vi "4461.Start.AI.vi"(6 "error in (no error)":errorcluster, 9 "Instrument.Lockin in":refnum<class "Instrument.Lockin.lvclass">) -> (0 "error out":errorcluster, 3 "Instrument.Lockin out":refnum<class "Instrument.Lockin.lvclass">)   [LabVIEW 2016, in "LockinDAQ.lvclass"]
uses:
  LockinDAQ.lvclass
  <resource>/objmgr/daqmx.rc
  <vilib>/DAQmx/read.llb/DAQmx Read (Analog 1D Wfm NChan NSamp).vi
  Instrument.Lockin/Instrument.Lockin.lvclass
  C:/Program Files (x86)/National Instruments/LabVIEW 2016/user.lib/LevyLab/Levylab Instruments/SMOs/Instrument/Instrument.lvclass
  C:/Program Files (x86)/National Instruments/LabVIEW 2016/user.lib/LevyLab/Levylab Instruments/SMOs/LevyLab/LevyLab.lvclass
  C:/Program Files (x86)/National Instruments/LabVIEW 2016/vi.lib/JKI/JKI SMO/SMO/SMO.lvclass
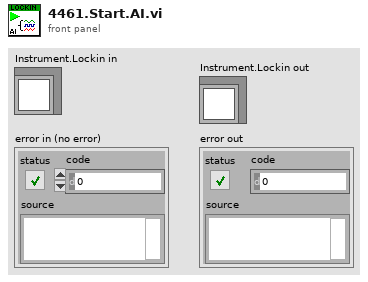
[diagram p1: front panel]
types:
  T1 = typedef "LockinDAQ.lvclass/DAQType-enum.ctl" = enum16{"None", "USB 4431", "PXI 446x"}
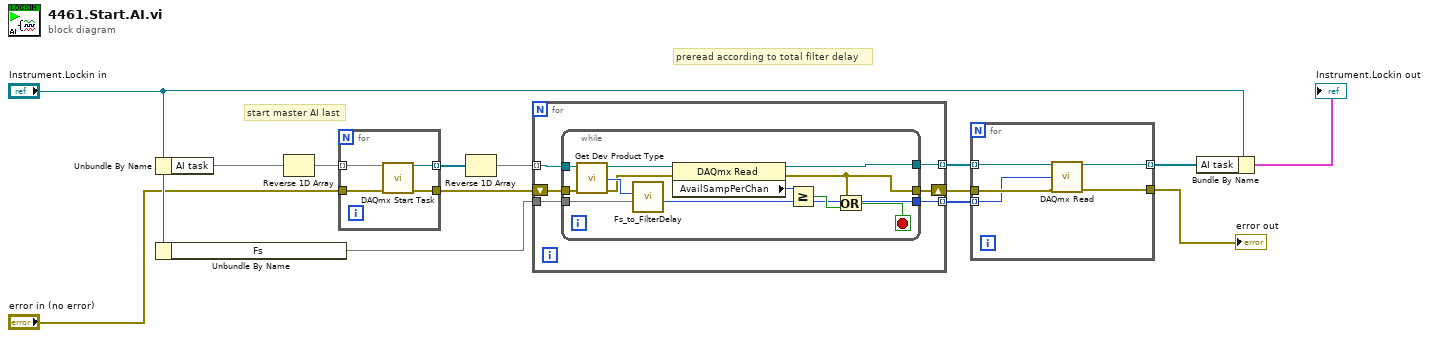
[diagram p0: block diagram]
diagram:
  # "preread according to total filter delay"
  # "start master AI last"
  n1 = Unbundle By Name("Instrument.Lockin in") -> ("AI task"=w12)
  n2 = Unbundle By Name("Instrument.Lockin in") -> ("Fs"=w8)
  n3 = Reverse 1D Array(array=w12) -> (reversed array=w11:void[])
  n4 = for {
    tunnel: w11 -> [w18] mode=indexing
    tunnel: "error in (no error)" -> [w17]
    tunnel: [w16] -> w10 mode=indexing
    tunnel: [w15] -> w9
    n5 = call <vilib>:"DAQmx Start Task.vi"("task/channels in"=w18, "error in"=w17) -> ("task out"=w16:refnum<k21>, "error out"=w15:errorcluster)  [unwired: 12 in]
  }
  n6 = Reverse 1D Array(array=w10) -> (reversed array=w1:refnum<k21>[])
  n7 = for {
    tunnel: w1 -> [w24] mode=indexing
    tunnel: w8 -> [w22]
    shift-right: [w21] -> w5
    shift-left: w9 -> [w23]
    tunnel: [w20] -> w7 mode=indexing
    tunnel: [w19] -> w6 mode=indexing
    n8 = while {
      tunnel: w24 -> [w36]
      tunnel: w23 -> [w35]
      tunnel: w22 -> [w34]
      tunnel: [w27] -> w21
      tunnel: [w26] -> w20
      tunnel: [w25] -> w19
      stop <- w29 stop-if-true
      n9 = call "Get Dev Product Type.vi"("error in (no error)"=w35, "Refnum in"=w36) -> ("error out"=w28:errorcluster, "DAQ Type"=w33:T1, "Refnum out"=w32:refnum<k21>)  [unwired: 6 in, 1 out]
      n10 = call "Fs_to_FilterDelay.vi"("Fs"=w34, "DAQ Type"=w33) -> ("Total Filter Delay (samples)"=w26:u32)  [unwired: 9 in]
      n11 = property class="DAQmx Read"(reference=w32, error in=w28) -> (reference out=w25:refnum<k21>, error out=w27:errorcluster, "AvailSampPerChan"=w31:u32)
      n12 = Greater Or Equal?(x=w31, y=w26) -> (x >= y?=w30:bool)
      n13 = Or(x=w27, y=w30) -> (x .or. y?=w29:bool)
    }
  }
  n14 = for {
    tunnel: w7 -> [w39] mode=indexing
    tunnel: w6 -> [w41] mode=indexing
    tunnel: w5 -> [w40]
    tunnel: [w38] -> w3
    tunnel: [w37] -> w4 mode=indexing
    n15 = call-poly <vilib>:"DAQmx Read.vi"("task/channels in"=w41, "number of samples per channel"=w39, "error in"=w40) -> ("task out"=w37:refnum<k21>, "error out"=w38:errorcluster)  [unwired: 10 in, 1 out]
  }
  "error out" <- w3
  n16 = Bundle By Name(cluster="Instrument.Lockin in", "AI task"=w4) -> (→"Instrument.Lockin out":cluster{})
